vi "FGV_PROXY_connection_indicators.vi"(4 "PLC_connections_indicator_global":refnum<vi>, 6 "SQL_connections_indicator_global":refnum<vi>, 7 "options":T1, 8 "error_in":errorcluster, 11 "status_array":bool[](array[boolean])) -> (0 "error_out":errorcluster)   [LabVIEW 2020]
uses:
  FGV_PROXY_connection_indicators.ctl
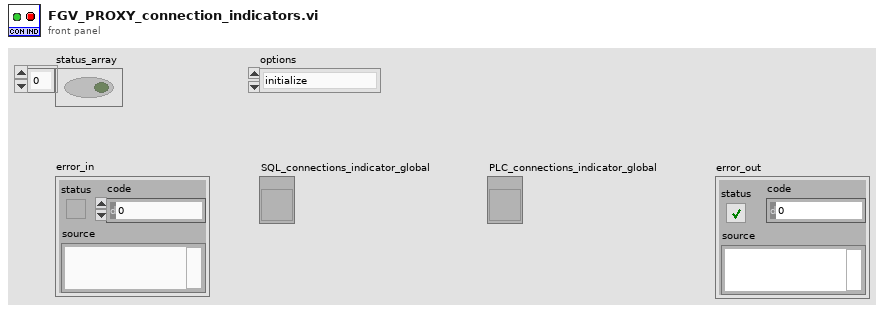
[diagram p1: front panel]
types:
  T1 = typedef "FGV_PROXY_connection_indicators.ctl" = enum16{"initialize", "SQL_conn_ind_update", "PLC_conn_ind_update"}
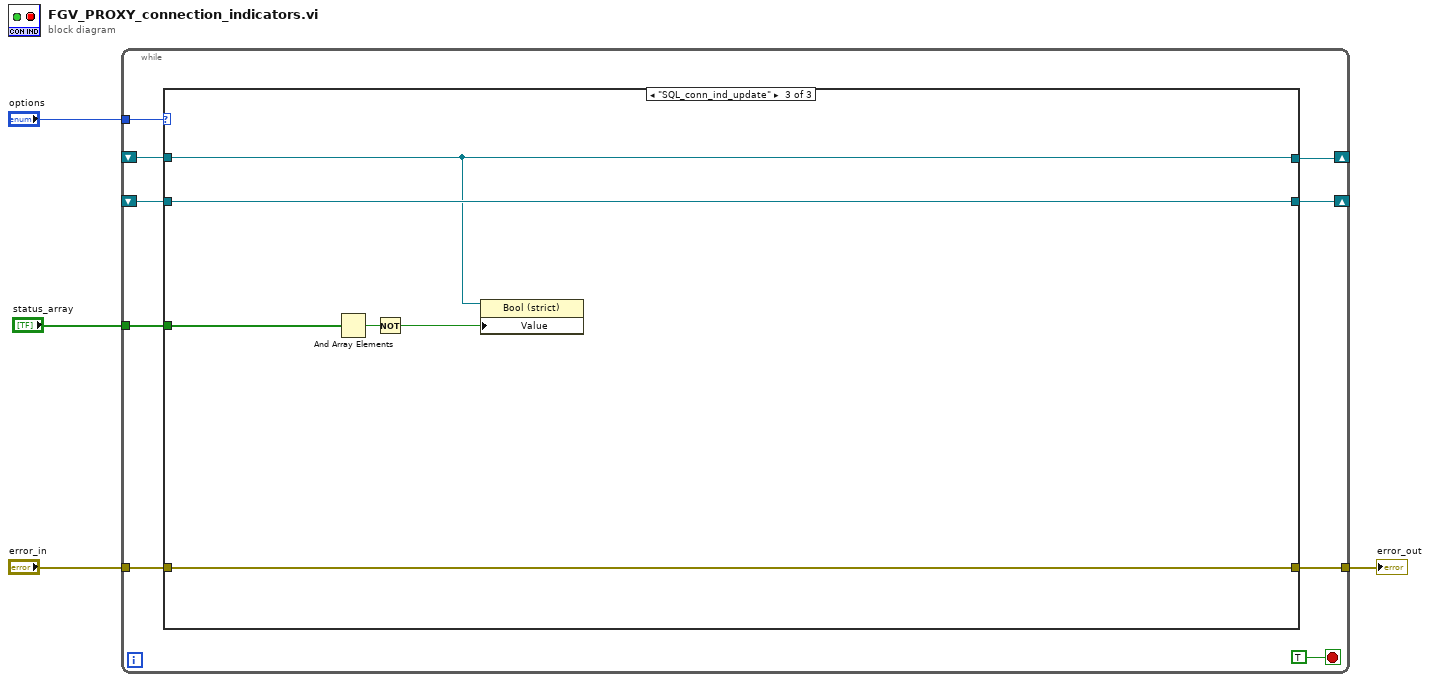
[diagram p0: block diagram]
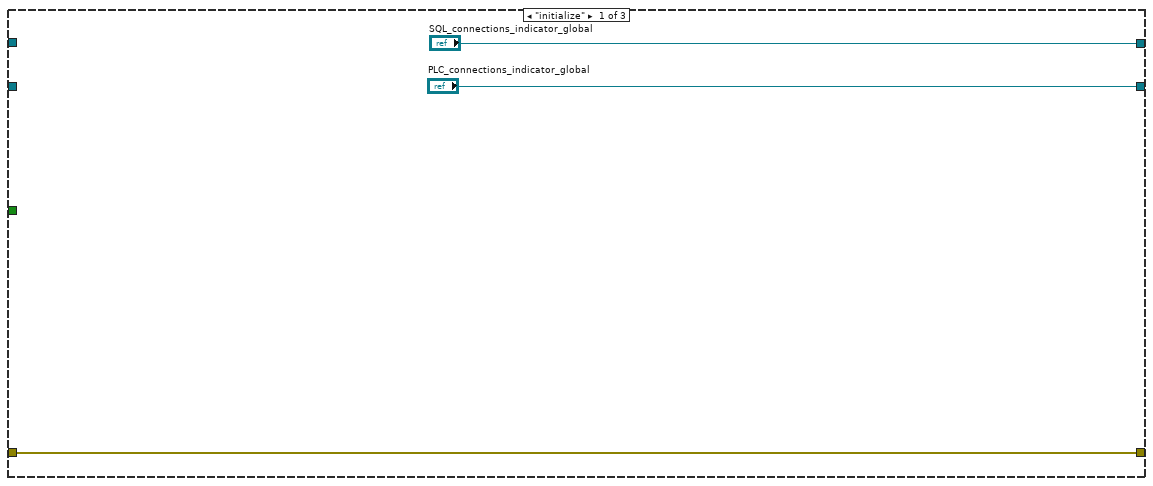
[diagram p2: hidden frame]
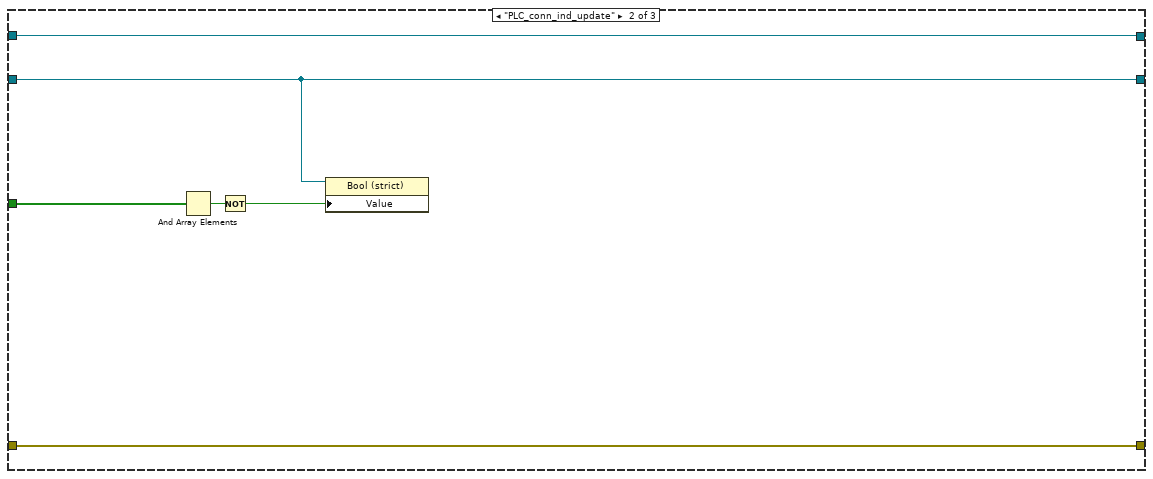
[diagram p3: hidden frame]
diagram:
  n1 = while {
    tunnel: "options" -> [w12]
    tunnel: [w11] -> w4
    tunnel: "error_in" -> [w10]
    shift-right: [w9] -> _
    shift-left: _ -> [w7]
    shift-right: [w8] -> _
    shift-left: _ -> [w6]
    tunnel: "status_array" -> [w5]
    stop <- TRUE stop-if-true
    n2 = case shown="\"SQL_conn_ind_update\"" w12 {
      tunnel: [w16 w22 w28] -> w11
      tunnel: w10 -> [w16 w22 w28]
      tunnel: ["SQL_connections_indicator_global" w20 w23] -> w9
      tunnel: ["PLC_connections_indicator_global" w18 w25] -> w8
      tunnel: w7 -> [_ w20 w23]
      tunnel: w6 -> [_ w18 w25]
      tunnel: w5 -> [_ w21 w27]
      frame "initialize" {
      }
      frame "PLC_conn_ind_update" {
        n3 = And Array Elements(Boolean array=w21) -> (logical AND=w19:bool)
        n4 = Not(x=w19) -> (.not. x?=w17:bool)
        n5 = property class="Bool (strict)"(reference=w18, "Value"=w17) -> ()  [unwired: 1 in, 2 out]
      }
      frame "SQL_conn_ind_update" {
        n6 = And Array Elements(Boolean array=w27) -> (logical AND=w26:bool)
        n7 = Not(x=w26) -> (.not. x?=w24:bool)
        n8 = property class="Bool (strict)"(reference=w23, "Value"=w24) -> ()  [unwired: 1 in, 2 out]
      }
    }
  }
  "error_out" <- w4
